vi "PH_IEEE1394Camera.evt call Set ROI.vi"(0 "i ref in":refnum<vi>, 2 "Instance":string, 3 "Top":u32, 4 "Bottom":u32, 5 "error in (no error)":errorcluster, 7 "Left":u32, 9 "Right":u32) -> (14 "i ref out":refnum<vi>, 19 "error out":errorcluster)   [LabVIEW 2014, in "PH_IEEE1394Camera.lvlib"]
doc: "This VI sends a simple call for SetROI."
uses:
  CS_Core/CSSystem/CoreLib/CoreLib.int 2 byte array.vi
  PH_IEEE1394Camera.lvlib
  CS_Core/CSSystem/CoreLib/CoreLib.lvlib
  CS_Core/BaseProcess/BaseProcess.lvlib
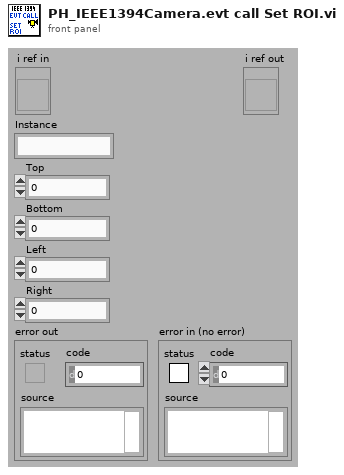
[diagram p1: front panel]
types:
  T1 = typedef "CoreDefs.rawDataType.ctl" = i8[]
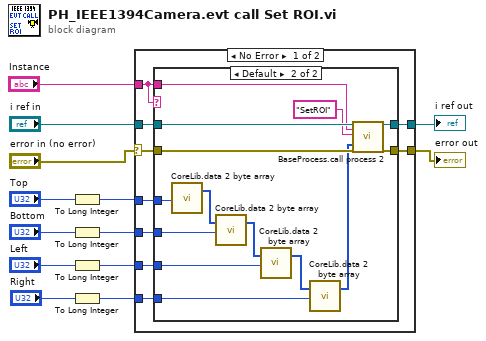
[diagram p0: block diagram]
diagram:
  n1 = To Long Integer(number="Top") -> (32bit integer=w7:i32)
  n2 = To Long Integer(number="Bottom") -> (32bit integer=w3:i32)
  n3 = To Long Integer(number="Left") -> (32bit integer=w2:i32)
  n4 = To Long Integer(number="Right") -> (32bit integer=w1:i32)
  n5 = case shown="No Error" "error in (no error)" {
    selector: "error in (no error)" -> [w19 w39]
    tunnel: [w22 w40] -> w11
    tunnel: [w21 w39] -> w10
    tunnel: "i ref in" -> [w20 w40]
    tunnel: "Instance" -> [w18 _]
    tunnel: w7 -> [w17 _]
    tunnel: w3 -> [w16 _]
    tunnel: w2 -> [w15 _]
    tunnel: w1 -> [w14 _]
    frame No Error {
      n6 = case shown="Default" w18 {
        tunnel: [w24 w38] -> w22
        tunnel: [w23 w37] -> w21
        tunnel: w20 -> [w24 w36]
        tunnel: w18 -> [_ w35]
        tunnel: w19 -> [w23 w33]
        tunnel: w17 -> [_ w32]
        tunnel: w16 -> [_ w31]
        tunnel: w15 -> [_ w29]
        tunnel: w14 -> [_ w27]
        frame "N/A" {
        }
        frame Default {
          n7 = call-poly "CoreLib.data 2 byte array.vi"("i32"=w32) -> ("byteArray out"=w30:T1)  [unwired: 18 in]
          n8 = call-poly "CoreLib.data 2 byte array.vi"("byteArray"=w30, "i32"=w31) -> ("byteArray out"=w28:T1)  [unwired: 17 in]
          n9 = call-poly "CoreLib.data 2 byte array.vi"("byteArray"=w28, "i32"=w29) -> ("byteArray out"=w26:T1)  [unwired: 17 in]
          n10 = call-poly "CoreLib.data 2 byte array.vi"("byteArray"=w26, "i32"=w27) -> ("byteArray out"=w25:T1)  [unwired: 17 in]
          n11 = call "BaseProcess.call process 2.vi"("i ref in"=w36, "Object"=w35, "Selector"="SetROI", "Data"=w25, "error in (no error)"=w33) -> ("i ref out"=w38:refnum<vi>, "error out"=w37:errorcluster)  [unwired: 13 in]
        }
      }
    }
    frame Error {
    }
  }
  "error out" <- w10
  "i ref out" <- w11
